vi "Pre Launch Init.vi"(11 "Controller in":refnum<class "Controller.lvclass">) -> (0 "error out":errorcluster, 3 "Controller out":refnum<class "Controller.lvclass">)   [LabVIEW 2016, in "Controller Actor.lvlib" / "Controller.lvclass"]
doc: "(<B>Filename</B>: Actor Framework.lvlib:Actor.lvclass:Pre Launch Init.vi)\n\nDefines behavior that occurs after the Launch Actor method is invoked but before the actor's Actor Core method begins running.\n\nThe Pre Launch Init method is guaranteed to finish before the Launch Actor method returns to its caller and before the actor itself receives any messages. Any references that the Pre Launch Init method obtains are guaranteed to have the same lifetime as the actor itself. Any errors that the Pre Launch Init method returns will abort the launch.\n\nBy default, this method does nothing. A descendant class may override it to define behavior."
uses:
  <userlib>/Common Components/Controller/Controller.lvclass
  <userlib>/Power-Requests-master/Power Availabilty Requests/Type Defs/Power Request Type.ctl
  <userlib>/Power-Requests-master/Power Availabilty Requests/Type Defs/Power Availiability Requests Functions.ctl
  <userlib>/Common Components/Controller/Controller.lvclass/Controller.ctl
  <vilib>/ActorFramework/Actor/Actor.lvclass
  <userlib>/Configuration Dialog Actor/Configuration.lvclass
  <userlib>/Power-Requests-master/Power Requests.lvlib
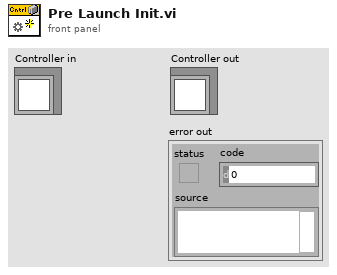
[diagram p1: front panel]
types:
  T1 = typedef "Power Requests.lvlib/Power Availiability Requests Functions.ctl" = enum32{"Power Create Request", "Power Set Request", "Power Clear Request", "Close Handle"}
  T2 = typedef "Power Requests.lvlib/Power Request Type.ctl" = enum32{"Power Request Display Required", "Power Request System Required", "Power Request Away Mode Required", "Power Request Execution Required"}
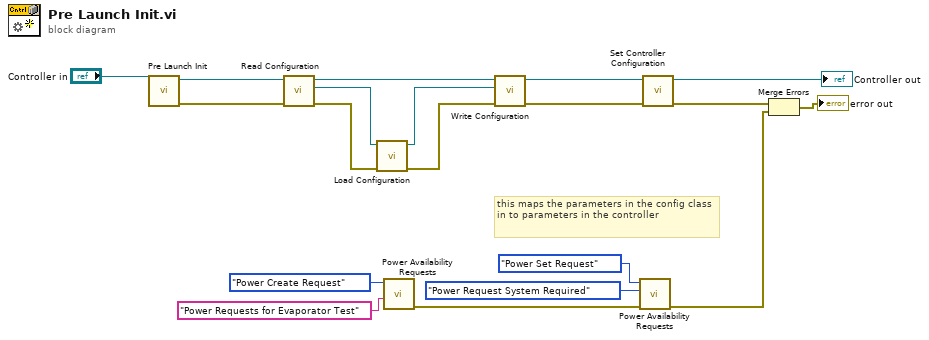
[diagram p0: block diagram]
diagram:
  # "this maps the parameters in the config class in to parameters in the controller"
  n1 = call-parent "Pre Launch Init.vi"("Actor in"="Controller in") -> ("error out"=w9:errorcluster, "Actor out"=w11:refnum<class "Controller.lvclass">)  [unwired: 9 in]
  n2 = call <userlib>:"Read Configuration.vi"("error in (no error)"=w9, "Controller in"=w11) -> ("error out"=w17:errorcluster, "Configuration.lvlib:Configuration.lvclass"=w18:refnum<class "Configuration.lvclass">, "Controller out"=w14:refnum<class "Controller.lvclass">)  [unwired: 7 in]
  n3 = call <userlib>:"Load Configuration.vi"("error in (no error)"=w17, "Configuration in"=w18) -> ("error out"=w15:errorcluster, "Configuration out"=w16:refnum<class "Configuration.lvclass">)  [unwired: 7 in, 1 out]
  n4 = call <userlib>:"Power Availability Requests.vi"("Simple Reason String"="Power Requests for Evaporator Test", "Power Availability Requests Functions"=Power_Availiability_Requests_Functions."Power Create Request") -> ("error out"=w5:errorcluster)  [unwired: 8 in, 1 out]
  n5 = call <userlib>:"Write Configuration.vi"("error in (no error)"=w15, "Configuration.lvlib:Configuration.lvclass"=w16, "Controller in"=w14) -> ("error out"=w12:errorcluster, "Controller out"=w13:refnum<class "Controller.lvclass">)  [unwired: 7 in]
  n6 = call <userlib>:"Power Availability Requests.vi"("error in (no error)"=w5, "Power Request Type"=Power_Request_Type."Power Request System Required", "Power Availability Requests Functions"=Power_Availiability_Requests_Functions."Power Set Request") -> ("error out"=w1:errorcluster)  [unwired: 7 in, 1 out]
  n7 = call-dynamic "Set Controller Configuration.vi"("error in (no error)"=w12, "Controller in"=w13) -> ("error out"=w8:errorcluster, "Controller out"=→"Controller out":refnum<class "Controller.lvclass">)  [unwired: 8 in]
  n8 = Merge Errors(w8, w1) -> (→"error out":errorcluster)
